vi "Retrieve Numeric String.vi"(11 "String in":string) -> (3 "Numeric String":string)   [LabVIEW 2018, in "Alicat Lib.lvlib" / "Alicat Device.lvclass"]
uses:
  Devices/Alicat/Session Based/Alicat Device.lvclass
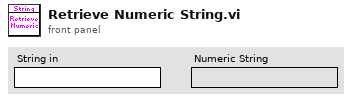
[diagram p1: front panel]
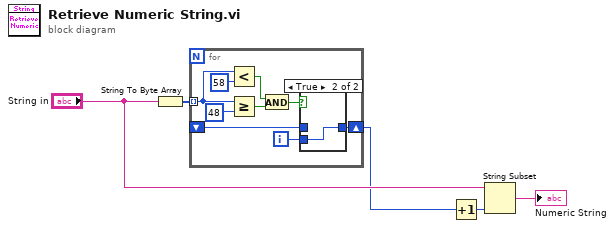
[diagram p0: block diagram]
diagram:
  n1 = String To Byte Array(string="String in") -> (unsigned byte array=w1:u8[])
  n2 = for {
    tunnel: w1 -> [w9] mode=indexing
    shift-right: [w13] -> w3
    shift-left: _ -> [w6]
    i -> [w14]
    n3 = Less?(x=w9, y=u8 58) -> (x < y?=w11:bool)
    n4 = Greater Or Equal?(x=w9, y=u8 48) -> (x >= y?=w10:bool)
    n5 = And(x=w11, y=w10) -> (x .and. y?=w7:bool)
    n6 = case shown="True" w7 {
      tunnel: w14 -> [_ w16]
      tunnel: [w15 w16] -> w13
      tunnel: w6 -> [w15 _]
      frame False {
      }
      frame True {
      }
    }
  }
  n7 = Increment(x=w3) -> (x+1=w2:i32)
  n8 = String Subset(string="String in", length (rest)=w2) -> (substring=→"Numeric String":string)  [unwired: 1 in]
